vi "CheesyDrive.vi"(6 "Quickturn":bool, 10 "Wheel":dbl(slide) scale=-1.0..1.0, 11 "Throttle":dbl(slide)=0.023622047244094488 scale=-1.0..1.0) -> (2 "Right PWM":dbl, 3 "Left PWM":dbl)   [LabVIEW 2017]
doc: "Implements CheesyDrive. CheesyDrive means that the turn joystick controls the radius of turning instead of the rate of turning. Also implements QuickStop and QuickTurn."
panel:
  in  "PointsTurn":cluster{"X":dbl, "Y":dbl}[](array[cluster])=[{"X"=0.0, "Y"=0.0}, {"X"=0.04, "Y"=0.0}, {"X"=0.041, "Y"=0.01}, {"X"=1.0, "Y"=1.0}]
  in  "PointsQuickTurn":cluster{"X":dbl, "Y":dbl}[](array[cluster])=[{"X"=0.0, "Y"=0.0}, {"X"=0.04, "Y"=0.0}, {"X"=0.041, "Y"=0.2}, {"X"=0.5, "Y"=0.5}, {"X"=1.0, "Y"=1.0}]
  in  "PointsThrottle":cluster{"X":dbl, "Y":dbl}[](array[cluster])=[{"X"=0.0, "Y"=0.0}, {"X"=0.025, "Y"=0.0}, {"X"=0.0251, "Y"=0.15}, {"X"=1.0, "Y"=1.0}]
  in  "CarLikeTurning":bool
  in  "QSMult":dbl=0.1
  in  "WheelNonLinearity":dbl=0.65
  in  "negInertiaScalar":dbl=3.0
  in  "Max dx/dt":dbl=9.0
  in  "alpha":dbl=0.1
  out "Waveform Chart":dbl(graph)
  in  "Sensitivty":dbl=1.0
  # "Enable to enable"
  # "(for quickstop decay)"
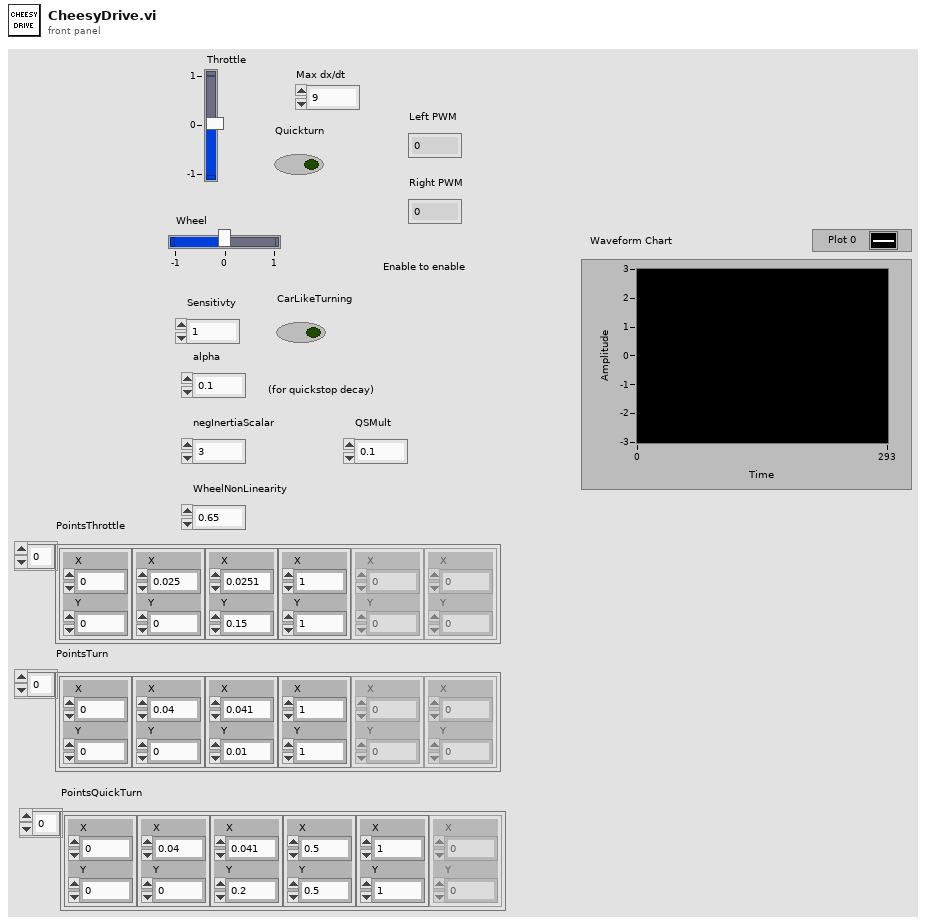
[diagram p1: front panel]
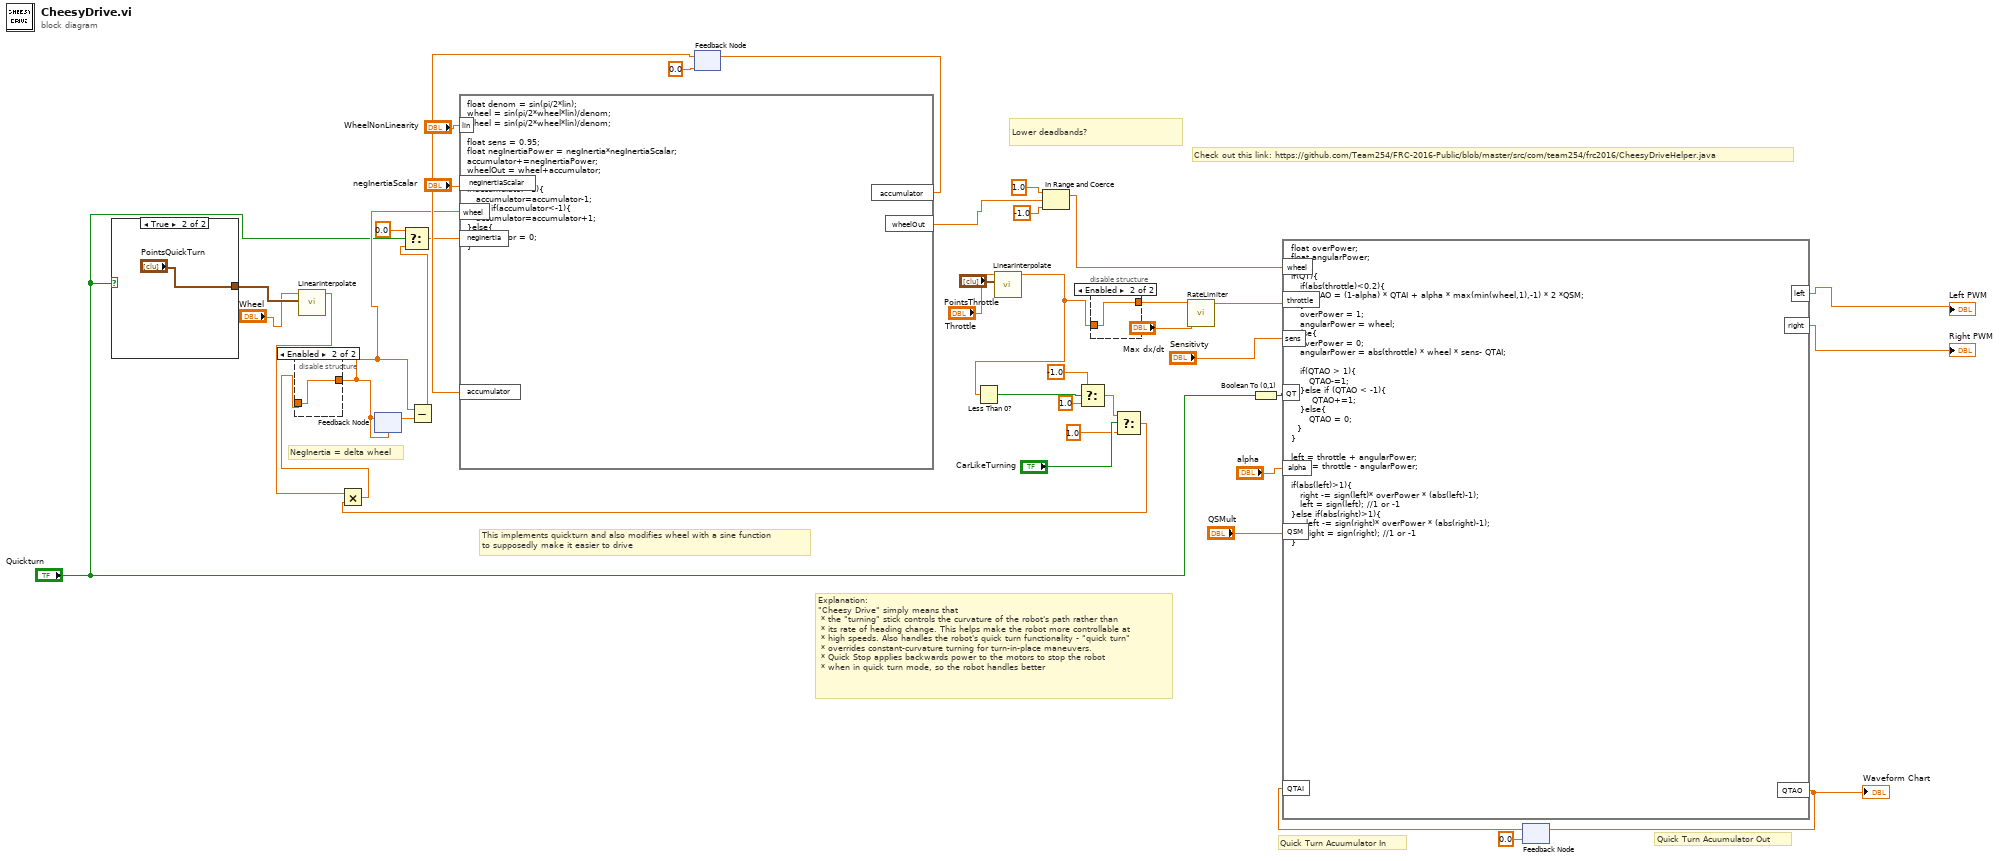
[diagram p0: block diagram]
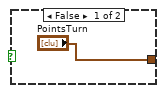
[diagram p2: hidden frame]
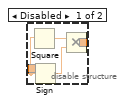
[diagram p3: hidden frame]
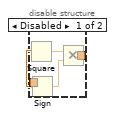
[diagram p4: hidden frame]
diagram:
  # "This implements quickturn and also modifies wheel with a sine function\nto supposedly make it easier to drive"
  # "Lower deadbands?"
  # "NegInertia = delta wheel"
  # "Explanation:\n\"Cheesy Drive\" simply means that\n * the \"turning\" stick controls the curvature of the robot's path rather than\n * its rate of heading change. This helps make the robot more controllable at\n * high speeds. Also handles the robot's quick turn functionality - \"quick turn\"\n * overrides constant-curvature turning for turn-in-place maneuvers.\n * Quick Stop applies backwards power to the motors to stop the robot\n * when in quick turn mode, so the robot handles better"
  # "Quick Turn Acuumulator Out"
  # "Quick Turn Acuumulator In"
  # "Check out this link: https://github.com/Team254/FRC-2016-Public/blob/master/src/com/team254/frc2016/CheesyDriveHelper.java"
  n1 = case shown="True" "Quickturn" {
    tunnel: ["PointsTurn" "PointsQuickTurn"] -> w7
    frame False {
    }
    frame True {
    }
  }
  n2 = call "LinearInterpolate.vi"("Points"=w7, "Value"="Wheel") -> ("Output"=w5:dbl)  [unwired: 9 in]
  n3 = feedback #1(0.0 ("Wheel")) -> (w29:dbl)
  n4 = call "LinearInterpolate.vi"("Points"="PointsThrottle", "Value"="Throttle") -> ("Output"=w8:dbl)  [unwired: 9 in]
  n5 = Less Than 0?(x=w8) -> (x < 0?=w19:bool)
  n6 = Select(t=-1.0, s=w19, f=1.0) -> (s? t:f=w13:dbl)
  n7 = disable-structure shown="Enabled" {
    disable-tunnel: [w45 w48] -> w35
    disable-tunnel: w8 -> [w44 w48]
    frame Disabled {
      n8 = Square(x=w44) -> (x^2=w47:dbl)
      n9 = Sign(1:w44) -> (0:w46:dbl)
      n10 = Multiply(x=w47, y=w46) -> (x*y=w45:dbl)
    }
    frame Enabled {
    }
  }
  n11 = Select(t=w13, s="CarLikeTurning", f=1.0) -> (s? t:f=w11:dbl)
  n12 = Multiply(x=w5, y=w11) -> (x*y=w16:dbl)
  n13 = disable-structure shown="Enabled" {
    disable-tunnel: w16 -> [w50 w53]
    disable-tunnel: [w49 w53] -> w15
    frame Disabled {
      n14 = Square(x=w50) -> (x^2=w52:dbl)
      n15 = Sign(1:w50) -> (0:w51:dbl)
      n16 = Multiply(x=w52, y=w51) -> (x*y=w49:dbl)
    }
    frame Enabled {
    }
  }
  n17 = feedback #2(w15) -> (w30:dbl)
  n18 = feedback-in #2(w15) -> ()
  n19 = Subtract(x=w15, y=w30) -> (x-y=w2:dbl)
  n20 = Select(t=0.0, s="Quickturn", f=w2) -> (s? t:f=w1:dbl)
  n21 = formula code="float denom = sin(pi/2*lin);\nwheel = sin(pi/2*wheel*lin)/denom;\nwheel = sin(pi/2*wheel*lin)/denom;\n\nfloat sens = 0.95;\nfloat negInertiaPower = negInertia*negInertiaScalar;\naccumulator+=negInertiaPower;\nwheelOut = wheel+accumulator;\n\nif(accumulator>1){\n   accumulator=accumulator-1;\n}else if(accumulator<-1){\n   accumulator=accumulator+1;\n}else{\naccumulator = 0;\n}"("wheel"=w15, "negInertia"=w1, "accumulator"=w29, "negInertiaScalar"="negInertiaScalar", "lin"="WheelNonLinearity") -> ("accumulator"=w27:dbl, "wheelOut"=w21:dbl)
  n22 = feedback-in #1(w27) -> ()
  n23 = In Range and Coerce(upper limit=1.0, x=w21, lower limit=-1.0) -> (coerced(x)=w22:dbl)  [unwired: 1 out]
  n24 = call "RateLimiter.vi"("Max dx/dt"="Max dx/dt", "Input"=w35) -> ("Output"=w34:dbl)  [unwired: 9 in]
  n25 = Boolean To (0,1)(Boolean="Quickturn") -> (0, 1=w39:i16)
  n26 = feedback #3(0.0 ("QTAccumulatorO")) -> (w37:dbl)
  n27 = formula code="float overPower;\nfloat angularPower;\n\nif(QT){\n   if(abs(throttle)<0.2){\n      QTAO = (1-alpha) * QTAI + alpha * max(min(wheel,1),-1) * 2 *QSM;\n   }\n   overPower = 1;\n   angularPower = wheel;\n}else{\n   overPower = 0;\n   angularPower = abs(throttle) * wheel * sens- QTAI;\n\n   if(QTAO > 1){\n      QTAO-=1;\n   }else if (QTAO < -1){\n       QTAO+=1;\n   }else{\n      QTAO = 0;\n  }\n}\n\nleft = throttle + angularPower;\nright = throttle - angularPower;\n\nif(abs(left)>1){\n   right -= sign(left)* overPower * (abs(left)-1);\n   left = sign(left); //1 or -1\n}else if(abs(right)>1){\n     left -= sign(right)* overPower * (abs(right)-1);\n     right = sign(right); //1 or -1 \n}"("wheel"=w22, "throttle"=w34, "sens"="Sensitivty", "QT"=w39, "alpha"="alpha", "QTAI"=w37, "QSM"="QSMult") -> ("left"=→"Left PWM":dbl, "right"=→"Right PWM":dbl, "QTAO"=w40:dbl)
  "Waveform Chart" <- w40
  n28 = feedback-in #3(w40) -> ()
